vi "Handle.vi"(11 "Base Event in":refnum<class "Base Event.lvclass">) -> (2 "Destroy?":bool, 3 "Base Event out":refnum<class "Base Event.lvclass">)   [LabVIEW 2021, in "jettl.lvlib" / "Base Event.lvlib" / "Base Event.lvclass"]
uses:
  Base Event.lvclass
  C:/git/jettl/src/jettl/Event/Event.lvclass
  Base Event.lvclass/Base Event.ctl
  State/State/State.lvclass
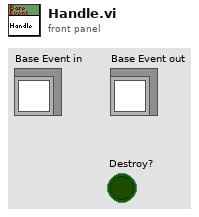
[diagram p1: front panel]
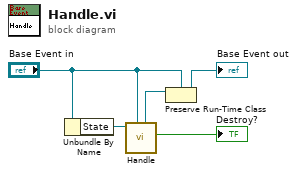
[diagram p0: block diagram]
diagram:
  n1 = Unbundle By Name("Base Event in") -> ("State"=w4:refnum<class "State.lvclass">)
  n2 = call-dynamic "Handle.vi"("Event jettl in"="Base Event in", "State in"=w4) -> ("Destroy?"=→"Destroy?":bool, "Event jettl out"=w2:refnum<class "Event.lvclass">)  [unwired: 8 in]
  n3 = Preserve Run-Time Class(object in=w2, 2:"Base Event in") -> (object out=→"Base Event out":refnum<class "Base Event.lvclass">)  [unwired: 1 in, 1 out]
